vi "Database.SaveResults.vi"(7 "Idx":i32, 8 "error in (no error)":errorcluster, 9 "Sets":T1, 10 "Data to export":T2, 11 "dbHandle":i32) -> (0 "error out":errorcluster, 1 "Export Time":timestamp, 2 "Data exported":T2, 3 "dbHandle out":i32)   [LabVIEW 2016]
uses:
  Cache/Cache.TestSteps.Fglb.ResultData.ctl
  ProdaNG/Controls/ProdaNG.ProcessResult.ctl
  ProdaNG/Controls/ProdaNG.ProcessStepResult.ctl
  ProdaNG/Controls/ProdaNG.TestStepResult.ctl
  ProdaNG/Controls/ProdaNG.TestValueResult.ctl
  Database.Data.Sets.ctl
  Tools/Translator/Translator.Message.ctl
  Tools/EventLog/EventLog.EventSource.ctl
  Tools/EventLog/EventLog.New(array).vi
  Global/ApplicationGlobal.vi
  Tools/EventLog/EventLog.Buffer.vi
  Tools/EventLog/EventLog.File.ReadWrite.vi
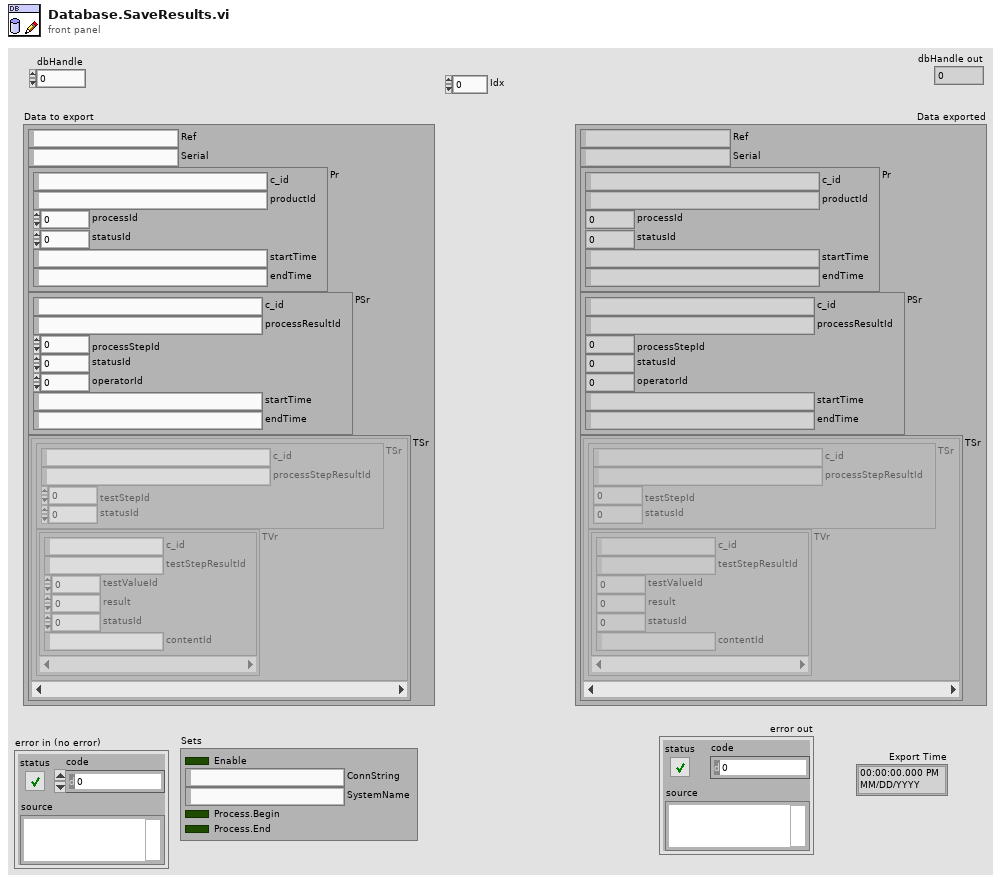
[diagram p1: front panel]
types:
  T1 = typedef "Database.Data.Sets.ctl" = cluster{"Enable":bool, "ConnString":string, "SystemName":string, "Process.Begin":bool, "Process.End":bool}
  T2 = typedef "Cache.TestSteps.Fglb.ResultData.ctl" = cluster{"Ref":string, "Serial":string, "Pr":T3, "PSr":T4, "TSr":cluster{"TSr":T5, "TVr":T6[]}[]}
  T3 = typedef "ProdaNG.ProcessResult.ctl" = cluster{"c_id":string, "productId":string, "processId":i32, "statusId":i32, "startTime":string, "endTime":string}
  T4 = typedef "ProdaNG.ProcessStepResult.ctl" = cluster{"c_id":string, "processResultId":string, "processStepId":i32, "statusId":i32, "operatorId":i32, "startTime":string, "endTime":string}
  T5 = typedef "ProdaNG.TestStepResult.ctl" = cluster{"c_id":string, "processStepResultId":string, "testStepId":i32, "statusId":i32}
  T6 = typedef "ProdaNG.TestValueResult.ctl" = cluster{"c_id":string, "testStepResultId":string, "testValueId":i32, "result":dbl, "statusId":i32, "contentId":string}
  T7 = typedef "EventLog.EventSource.ctl" = enum16{"All", "Gui", "PLC1", "PLC2", "PLC3", "DB", "DB01", "DB02", "DB03", "DB04", "DB05", "DB06", "DB07", "DB08", "DB09", "DB10", "DB11", "DB12", "DB13", "DB14", "DB15", "DB16"}
  T8 = typedef "Translator.Message.ctl" = enum16{"-", "Event confirmed", "Log out", "Log in", "Shutdown", "Cancel", "Start", "Continue", "Stop", "On", "Off", "OK", "NOK", "NOK %s", "This", "Prev", "Home", "Work", "In progress...", "Missing", "Empty", "Hardware failure", "Initial", "Error %d >> %s", "Error %d >> %s >> %s", "Starting %s", "Quitting %s", "Configured", "Initializing", "Quitting", "Loading", "Running %s", "Stopped", "Summary", "Do you want to continue?", "Do you want to exit?", "Log out?", "System", "All", "IDLE", "Translating...%s", "Not found", "Alarm %s", "Run", "Skip", "Abort", "Repeat", "Please wait...", "Database disconnected", "Login to database successful", "Login to database failed: %d; %s", "Get process step data for %s", "Changeover off", "Changeover into %s", "Product %s | %s found in cache with status %d at previous station", "Product %s | %s found in database with status %d at previous station", "Product %s | %s not found in cache at previous station", "Product %s | %s not found in database at previous station", "Product %s | %s found in cache with status %d at this station (%d repetion)", "Product %s | %s found in database with status %d at this station (%d repetition)", "Product %s | %s not found in cache at this station", "Product %s | %s not found in database at this station", "Product %s | %s found in cache for component %s | %s", "Product %s | %s found in database for component %s | %s", "Product not found in cache for component %s | %s", "Product not found in database for component %s | %s", "Product %s | %s connected with component %s | %s (cache)", "Product %s | %s connected with component %s | %s (database)", "New data for %s | %s (cache)", "New data for %s | %s (database)", "Msg %d >> %s", "PLC LifeBit Failure", "Reconnecting DB", "Reconnecting PLC"}
  T9 = typedef "ProdaNG.Identification.ctl" = cluster{"processId":i32, "systemId":i32, "processStepId":i32, "wabcoPartId":i32}
  T10 = typedef "ProdaNG.Product.ctl" = cluster{"c_id":string, "wabcoPartId":i32, "serialNumber":string, "comment":string, "individual":i32, "crProcessStepId":i32, "mdProcessStepId":i32, "crTime":string, "mdTime":string}
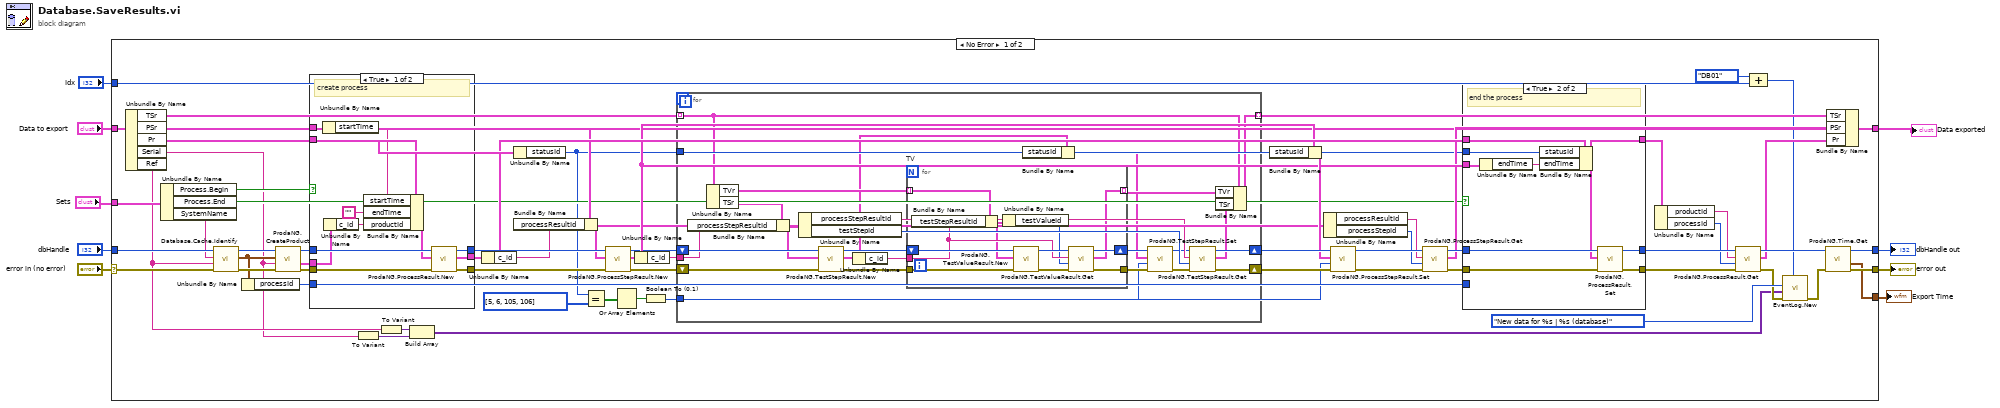
[diagram p0: block diagram]
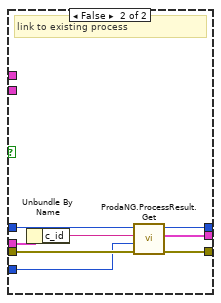
[diagram p2: hidden frame]
diagram:
  n1 = case shown="No Error" "error in (no error)" {
    selector: "error in (no error)" -> [w31 w144]
    tunnel: [w68 w144] -> w9
    tunnel: [w67 w143] -> w7
    tunnel: "dbHandle" -> [w27 w143]
    tunnel: [w66 _] -> w5
    tunnel: "Data to export" -> [w37 w142]
    tunnel: [w38 w142] -> w3
    tunnel: "Sets" -> [w34 _]
    tunnel: "Idx" -> [w18 _]
    frame No Error {
      n2 = Unbundle By Name(w37) -> ("TSr"=w69:cluster{"TSr":T5, "TVr":T6[]}[], "PSr"=w36:T4, "Pr"=w63:T3, "Serial"=w16:string, "Ref"=w17:string)
      n3 = Unbundle By Name(w34) -> ("Process.Begin"=w33:bool, "Process.End"=w32:bool, "SystemName"=w26:string)
      n4 = call "Database.Cache.Identify.vi"("error in (no error)"=w31, "Variant"=w17, "SystemName"=w26, "DB Handle in"=w27) -> ("error out"=w30:errorcluster, "SytemID"=w29:T9, "DB Handle out"=w28:i32)  [unwired: 5 in]
      n5 = Unbundle By Name(w29) -> ("processId"=w35:i32)
      n6 = call "ProdaNG.CreateProduct.vi"("error in (no error)"=w30, "serialNumber"=w16, "ID"=w29, "dbHandle"=w28) -> ("error out"=w64:errorcluster, "Product out"=w62:T10, "dbHandle out"=w65:i32)  [unwired: 5 in]
      n7 = case shown="True" w33 {
        tunnel: w65 -> [w121 w128]
        tunnel: w64 -> [w120 w129]
        tunnel: w63 -> [w119 _]
        tunnel: [w117 w127] -> w60
        tunnel: [w116 w125] -> w61
        tunnel: [w115 w126] -> w59
        tunnel: w62 -> [w114 w124]
        tunnel: w36 -> [w111 _]
        tunnel: w35 -> [_ w122]
        frame True {
          # "create process"
          n8 = Unbundle By Name(w111) -> ("startTime"=w110:string)
          n9 = Unbundle By Name(w114) -> ("c_id"=w113:string)
          n10 = Bundle By Name(cluster=w119, "startTime"=w110, "endTime"="", "productId"=w113) -> (w118:T3)
          n11 = call "ProdaNG.ProcessResult.New.vi"("error in (no error)"=w120, "ProcessResult"=w118, "dbHandle"=w121) -> ("error out"=w117:errorcluster, "ProcessResult out"=w115:T3, "dbHandle"=w116:i32)  [unwired: 6 in]
        }
        frame False {
          # "link to existing process"
          n12 = Unbundle By Name(w124) -> ("c_id"=w123:string)
          n13 = call "ProdaNG.ProcessResult.Get.vi"("error in (no error)"=w129, "processId"=w122, "productId"=w123, "dbHandle"=w128) -> ("error out"=w127:errorcluster, "ProcessResult"=w126:T3, "dbHandle out"=w125:i32)  [unwired: 4 in, 1 out]
        }
      }
      n14 = To Variant(anything=w16) -> (Variant=w25:variant)
      n15 = To Variant(anything=w17) -> (Variant=w24:variant)
      n16 = Build Array(w24, w25) -> (w15:variant[])
      n17 = Unbundle By Name(w59) -> ("c_id"=w44:string)
      n18 = Unbundle By Name(w63) -> ("statusId"=w12:i32)
      n19 = Bundle By Name(cluster=w36, "processResultId"=w44) -> (w50:T4)
      n20 = Equal?(x=w12, y=u8[] [5, 6, 105, 106]) -> (x = y?=w14:bool[])
      n21 = call "ProdaNG.ProcessStepResult.New.vi"("error in (no error)"=w60, "ProcessStepResult"=w50, "dbHandle"=w61) -> ("error out"=w56:errorcluster, "ProcessStepResult out"=w58:T4, "dbHandle"=w57:i32)  [unwired: 6 in]
      n22 = Or Array Elements(Boolean array=w14) -> (logical OR=w11:bool)
      n23 = Unbundle By Name(w58) -> ("c_id"=w73:string)
      n24 = Boolean To (0,1)(Boolean=w11) -> (0, 1=w10:i16)
      n25 = for "TS" {
        tunnel: w73 -> [w88]
        shift-right: [w89] -> w71
        shift-left: w57 -> [w97]
        tunnel: w69 -> [w91] mode=indexing
        tunnel: [w84] -> w55 mode=indexing
        shift-right: [w90] -> w72
        shift-left: w56 -> [w98]
        tunnel: w12 -> [w77]
        tunnel: w10 -> [w74]
        n26 = Unbundle By Name(w91) -> ("TVr"=w96:T6[], "TSr"=w78:T5)
        n27 = Bundle By Name(cluster=w78, "processStepResultId"=w88) -> (w87:T5)
        n28 = Unbundle By Name(w87) -> ("processStepResultId"=w83:string, "testStepId"=w86:i32)
        n29 = call "ProdaNG.TestStepResult.New.vi"("error in (no error)"=w98, "TestStepResult"=w87, "dbHandle"=w97) -> ("error out"=w94:errorcluster, "TestStepResult out"=w76:T5, "dbHandle"=w95:i32)  [unwired: 6 in]
        n30 = Unbundle By Name(w76) -> ("c_id"=w93:string)
        n31 = for "TV" {
          tunnel: w94 -> [w109]
          tunnel: [w101] -> w81
          tunnel: w93 -> [w104]
          tunnel: w96 -> [w106] mode=indexing
          shift-right: [w100] -> w82
          shift-left: w95 -> [w108]
          tunnel: [w99] -> w92 mode=indexing
          n32 = Bundle By Name(cluster=w106, "testStepResultId"=w104) -> (w103:T6)
          n33 = Unbundle By Name(w103) -> ("testValueId"=w102:i32)
          n34 = call "ProdaNG.TestValueResult.New.vi"("error in (no error)"=w109, "TestValueResult"=w103, "dbHandle"=w108) -> ("error out"=w105:errorcluster, "dbHandle"=w107:i32)  [unwired: 7 in]
          n35 = call "ProdaNG.TestValueResult.Get.vi"("error in (no error)"=w105, "testValueId"=w102, "testStepResultId"=w104, "dbHandle"=w107) -> ("error out"=w101:errorcluster, "TestValueResult"=w99:T6, "dbHandle"=w100:i32)  [unwired: 5 in]
        }
        n36 = Bundle By Name(cluster=w76, "statusId"=w77) -> (w75:T5)
        n37 = call "ProdaNG.TestStepResult.Set.vi"("error in (no error)"=w81, "isRepeat (0)"=w74, "TestStepResult"=w75, "dbHandle"=w82) -> ("error out"=w79:errorcluster, "dbHandle"=w80:i32)  [unwired: 6 in]
        n38 = call "ProdaNG.TestStepResult.Get.vi"("error in (no error)"=w79, "testStepId"=w86, "processStepResulttId"=w83, "dbHandle"=w80) -> ("error out"=w90:errorcluster, "TestStepResult"=w85:T5, "dbHandle out"=w89:i32)  [unwired: 4 in, 1 out]
        n39 = Bundle By Name(cluster=w91, "TVr"=w92, "TSr"=w85) -> (w84:cluster{"TSr":T5, "TVr":T6[]})
      }
      n40 = Bundle By Name(cluster=w58, "statusId"=w12) -> (w70:T4)
      n41 = Unbundle By Name(w50) -> ("processResultId"=w43:string, "processStepId"=w49:i32)
      n42 = call "ProdaNG.ProcessStepResult.Set.vi"("error in (no error)"=w72, "isRepeat (-1: auto)"=w10, "ProcessStepResult"=w70, "dbHandle"=w71) -> ("error out"=w54:errorcluster, "dbHandle"=w53:i32)  [unwired: 6 in]
      n43 = call "ProdaNG.ProcessStepResult.Get.vi"("error in (no error)"=w54, "processStepId"=w49, "processResultId"=w43, "dbHandle"=w53) -> ("error out"=w51:errorcluster, "ProcessStepResult"=w48:T4, "dbHandle out"=w52:i32)  [unwired: 4 in, 1 out]
      n44 = case shown="True" w32 {
        tunnel: w52 -> [w132 w141]
        tunnel: w51 -> [w131 w140]
        tunnel: [w132 w134] -> w47
        tunnel: [w131 w135] -> w46
        tunnel: w12 -> [_ w138]
        tunnel: w59 -> [w130 w137]
        tunnel: w58 -> [_ w136]
        tunnel: [w130 w133] -> w42
        tunnel: w35 -> [_ _]
        frame False {
        }
        frame True {
          # "end the process"
          n45 = Unbundle By Name(w136) -> ("endTime"=w139:string)
          n46 = Bundle By Name(cluster=w137, "statusId"=w138, "endTime"=w139) -> (w133:T3)
          n47 = call "ProdaNG.ProcessResult.Set.vi"("error in (no error)"=w140, "ProcessResult"=w133, "dbHandle"=w141) -> ("error out"=w135:errorcluster, "dbHandle"=w134:i32)  [unwired: 7 in]
        }
      }
      n48 = Unbundle By Name(w42) -> ("productId"=w41:string, "processId"=w40:i32)
      n49 = call "ProdaNG.ProcessResult.Get.vi"("error in (no error)"=w46, "processId"=w40, "productId"=w41, "dbHandle"=w47) -> ("error out"=w20:errorcluster, "ProcessResult"=w39:T3, "dbHandle out"=w45:i32)  [unwired: 4 in, 1 out]
      n50 = Compound Arithmetic op=ADD(EventLog.EventSource."DB01" ("Source (All)"), w18) -> (w21:i32)
      n51 = call-poly "EventLog.New.vi"("Source (All)"=w21, "error in (no error)"=w20, "Arguments"=w15, "Message (-)"=Translator.Message."New data for %s | %s (database)") -> ("error out"=w19:errorcluster)  [unwired: 6 in, 1 out]
      n52 = call "ProdaNG.Time.Get.vi"("error in"=w19, "dbHandleIn"=w45) -> ("error out"=w68:errorcluster, "time"=w66:timestamp, "dbHandle"=w67:i32)  [unwired: 5 in, 1 out]
      n53 = Bundle By Name(cluster=w37, "TSr"=w55, "PSr"=w48, "Pr"=w39) -> (w38:T2)
    }
    frame Error {
    }
  }
  "error out" <- w9
  "dbHandle out" <- w7
  "Export Time" <- w5
  "Data exported" <- w3
